vi "build_rs232_command_packet.vi"(9 "Data bytes":u8[](array[numeric]), 10 "Command byte":u8) -> (2 "Command packet":string)   [LabVIEW 2018]
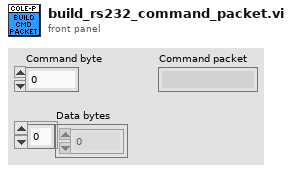
[diagram p1: front panel]
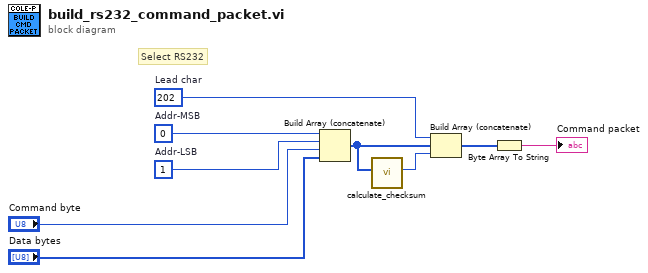
[diagram p0: block diagram]
diagram:
  w2 = u8 1  # Addr-LSB
  w1 = u8 0  # Addr-MSB
  w4 = u8 202  # Lead char
  # "Select RS232"
  n1 = Build Array (concatenate)(w1, w2, "Command byte", "Data bytes") -> (w5:u8[])
  n2 = call "calculate_checksum.vi"("Byte array"=w5) -> ("Checksum"=w6:u8)  [unwired: 10 in]
  n3 = Build Array (concatenate)(w4, w5, w6) -> (w9:u8[])
  n4 = Byte Array To String(unsigned byte array=w9) -> (string=→"Command packet":string)
